vi "Actor Core.vi"(8 "error in":errorcluster, 11 "New Project Wizard in":refnum<class "Update Project Wizard.lvclass">) -> (0 "error out":errorcluster, 3 "Actor out":refnum<class "Actor.lvclass">)   [LabVIEW 2013, in "SET Project Editor.lvlib" / "Update Project Wizard.lvclass"]
doc: "(<B>Filename</B>: Actor Framework.lvlib:Actor.lvclass:Actor Core.vi)\n\nReceives messages to the actor, reacts to them, and initiates any error handling that may shut the actor down.\n\nDescendant classes may override this VI to append parallel tasks for the actor to complete while it handles messages. Overrides use the Call Parent Method node."
uses:
  Update Project Wizard.lvclass
  <vilib>/ActorFramework/Actor/Actor.lvclass
  <vilib>/ActorFramework/Actor/Actor.lvclass/Actor.ctl
  <vilib>/ActorFramework/Message Enqueuer/Message Enqueuer.lvclass/Message Enqueuer.ctl
  Update Project Wizard.lvclass/Update Project Wizard.ctl
  lib/printf/messages/General/LV_Printf Msg.lvclass/LV_Printf Msg.ctl
  UI Wizard/UI Wizard.lvclass
  lib/printf/messages/General/Read Message.vi
  <vilib>/ActorFramework/Message Enqueuer/Init from Existing Queue.vi
  <vilib>/ActorFramework/Message Enqueuer/Enqueue.vi
  <vilib>/ActorFramework/Message Priority Queue/Priority Enqueue.vi
  <vilib>/ActorFramework/Message Enqueuer/Message Enqueuer.lvclass
  <vilib>/ActorFramework/Stop Msg/Stop Msg.lvclass
  UI Wizard Messages/Extract Project Strings Msg/Extract Project Strings Msg.lvclass
  UI Wizard Messages/Apply Changes Msg/Apply Changes Msg.lvclass
  lib/printf/Core/LV_Printf Core.lvclass
  lib/printf/messages/General/LV_Printf Msg.lvclass
panel:
  in  "Tab Control":enum32{"Page 1", "Page 2"}(tab)
  in  "Next1":bool
  out "ProjectName":string
  in  "Cancel1":bool
  in  "VI Selector":i32(listbox)
  in  "RTM Selector":i32(listbox)
  out "Status":string
  in  "Prev2":bool
  in  "Finish":bool
  # "Update Project Wizard"
  # "Select VIs"
  # "Select Run-Time Menus"
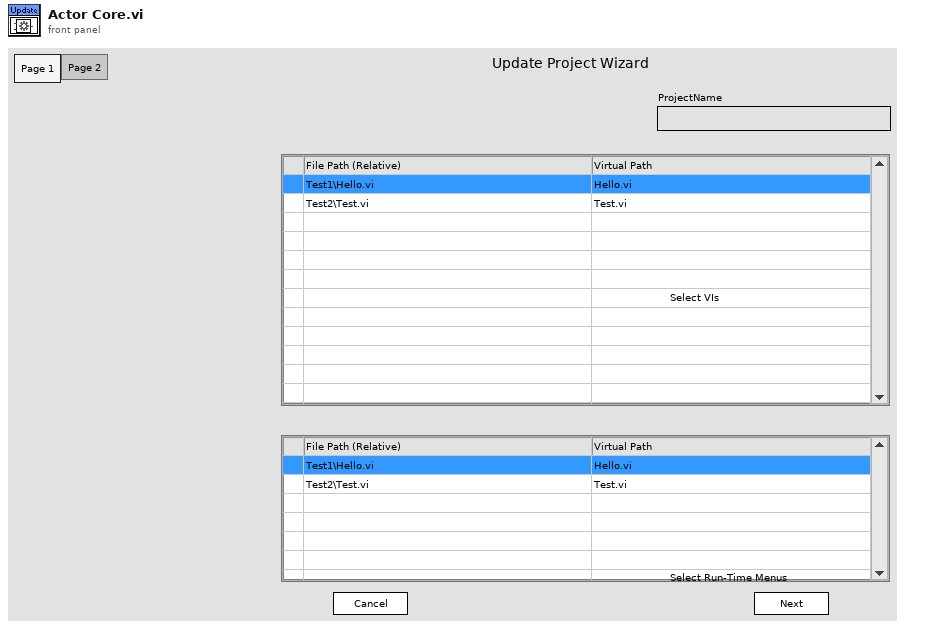
[diagram p1: front panel]
types:
  T1 = typedef "LVPoint32TypeDef.ctl" = cluster{"Horizontal":i32, "Vertical":i32}
  T2 = typedef "LVRowAndColumnTypeDef.ctl" = cluster{"Row":i32, "Column":i32}
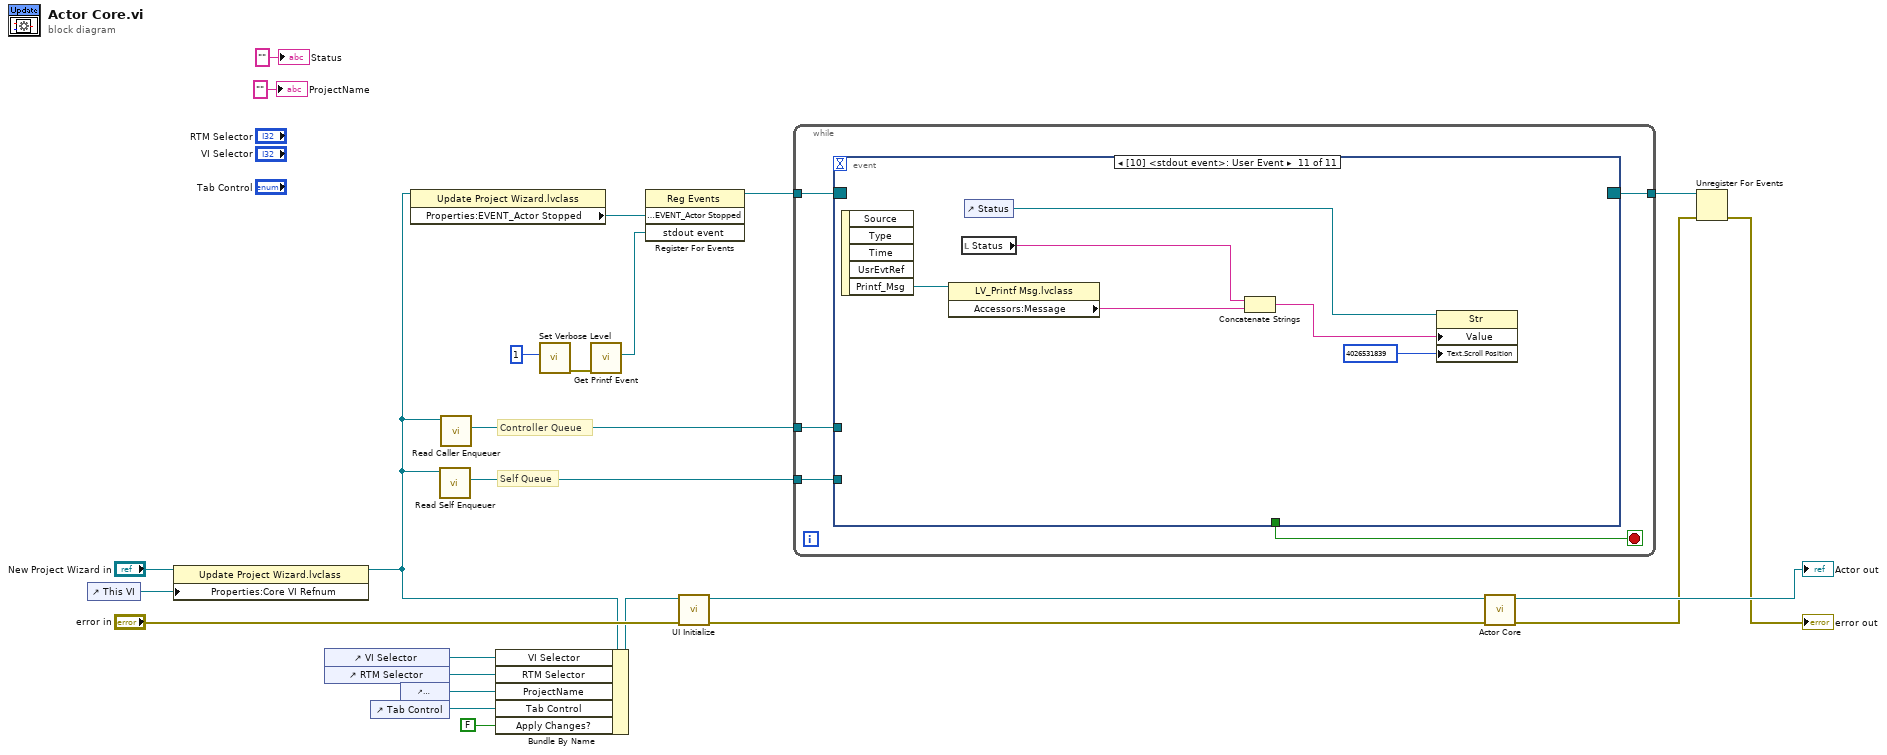
[diagram p0: block diagram]
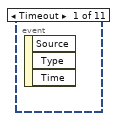
[diagram p2: hidden frame]
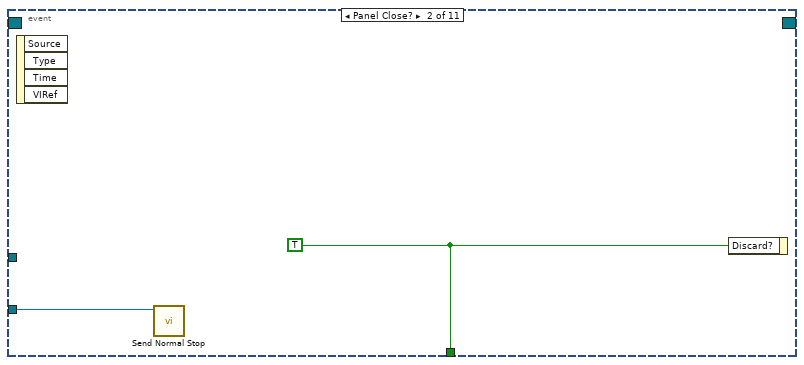
[diagram p3: hidden frame]
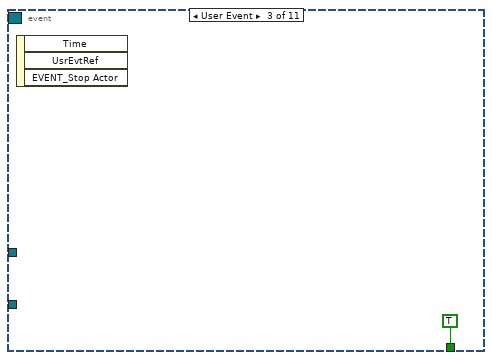
[diagram p4: hidden frame]
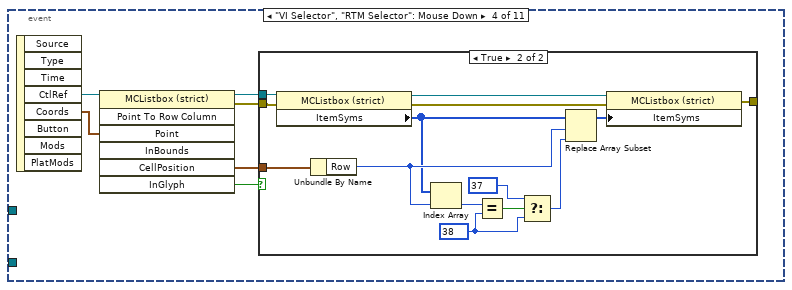
[diagram p5: hidden frame]
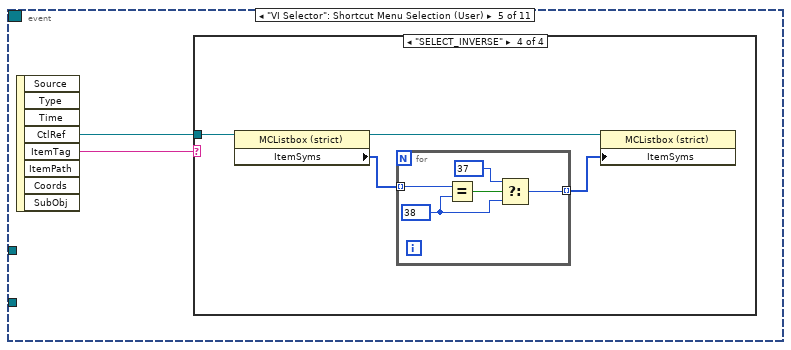
[diagram p7: hidden frame]
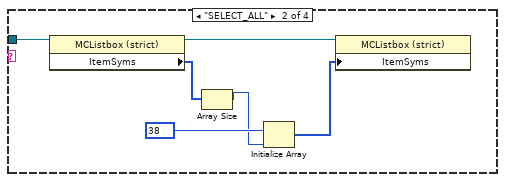
[diagram p9: hidden frame]
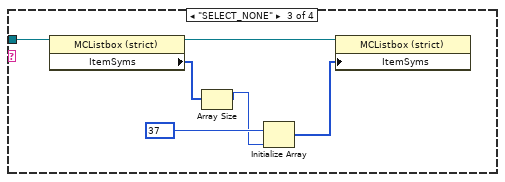
[diagram p10: hidden frame]
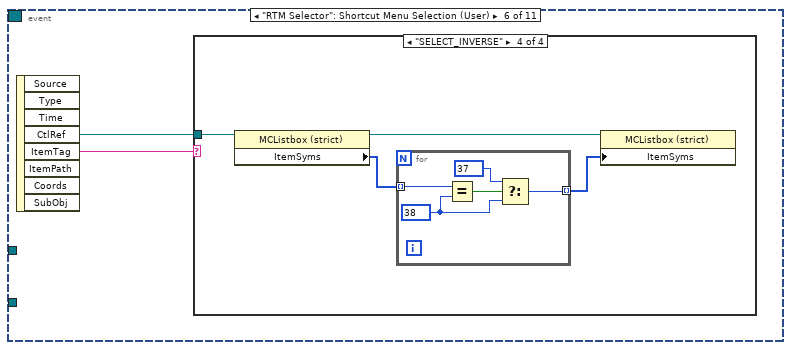
[diagram p11: hidden frame]
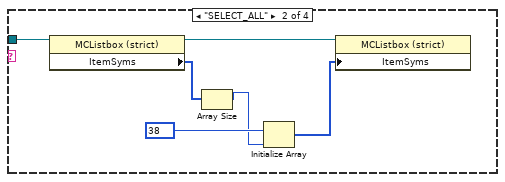
[diagram p13: hidden frame]
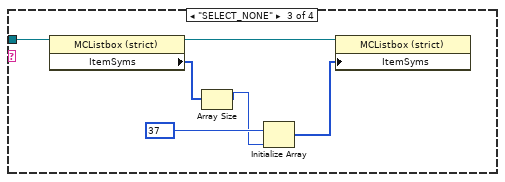
[diagram p14: hidden frame]
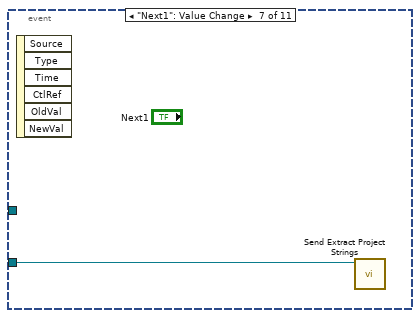
[diagram p15: hidden frame]
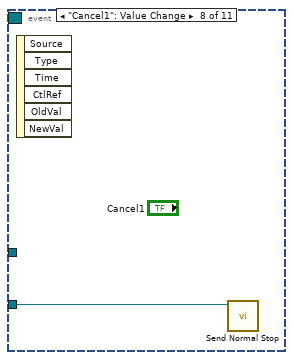
[diagram p16: hidden frame]
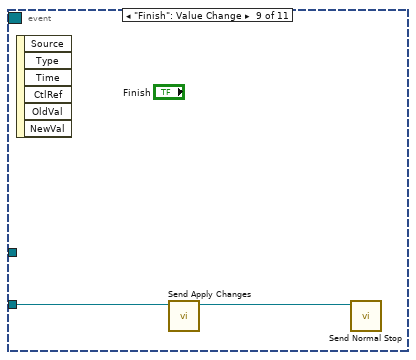
[diagram p17: hidden frame]
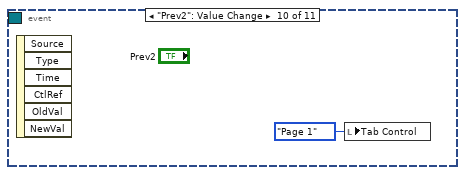
[diagram p18: hidden frame]
diagram:
  # "Controller Queue"
  # "Self Queue"
  n1 = control-ref of="This VI"() -> (w17:refnum<vi>)
  n2 = property class="Update Project Wizard.lvclass"(reference="New Project Wizard in", "Properties:Core VI Refnum"=w17) -> (reference out=w9:refnum<class "Update Project Wizard.lvclass">)  [unwired: 1 in, 1 out]
  n3 = control-ref of="VI Selector"() -> (w7:refnum<vi>)
  n4 = control-ref of="RTM Selector"() -> (w6:refnum<vi>)
  n5 = control-ref of="Tab Control"() -> (w4:refnum<vi>)
  n6 = control-ref of="ProjectName"() -> (w5:refnum<vi>)
  n7 = property class="Update Project Wizard.lvclass"(reference=w9) -> ("Properties:EVENT_Actor Stopped"=w24:refnum<user-event>)  [unwired: 1 in, 2 out]
  n8 = call <vilib>:"Read Self Enqueuer.vi"("Actor"=w9) -> ("Self Enqueuer"=w22:refnum<class "Message Enqueuer.lvclass">)  [unwired: 10 in]
  n9 = call <vilib>:"Read Caller Enqueuer.vi"("Actor"=w9) -> ("Caller Enqueuer"=w23:refnum<class "Message Enqueuer.lvclass">)  [unwired: 10 in]
  n10 = Bundle By Name(cluster=w9, "VI Selector"=w7, "RTM Selector"=w6, "ProjectName"=w5, "Tab Control"=w4, "Apply Changes?"=FALSE) -> (w8:refnum<class "Update Project Wizard.lvclass">)
  n11 = call "Set Verbose Level.vi"("Verbose Level"=1) -> ("error out"=w11:errorcluster)  [unwired: 10 in]
  n12 = call "Get Printf Event.vi"("error in (no error)"=w11) -> ("stdout event"=w10:refnum<user-event>)  [unwired: 8 in, 2 out]
  n13 = register-events(w24, w10) -> (reference out=w12:refnum<event-registration>)  [unwired: 2 in, 1 out]
  n14 = call-dynamic "UI Initialize.vi"("error in (no error)"="error in", "New Project Wizard in"=w8) -> ("error out"=w15:errorcluster, "New Project Wizard out"=w16:refnum<class "Update Project Wizard.lvclass">)  [unwired: 8 in]
  n15 = while {
    tunnel: w12 -> [w29]
    tunnel: [w28] -> w21
    tunnel: w22 -> [w27]
    tunnel: w23 -> [w26]
    stop <- w30 stop-if-true
    n16 = event shown="[10] <stdout event>: User Event" {
      selector: w29 -> [_ _ _ _ _ _ _ _ _ _ _]
      dyn-events: [_ _ _ _ _ _ _ _ _ _ _] -> w28
      timeout: _ -> [_ _ _ _ _ _ _ _ _ _ _]
      tunnel: [_ w32 TRUE ("Discard?") _ _ _ _ _ _ _ _] -> w30
      tunnel: w27 -> [_ w31 _ _ _ _ w101 w102 w104 _ _]
      tunnel: w26 -> [_ _ _ _ _ _ _ _ _ _ _]
      event Timeout {
        n17 = event-data() -> ()  [unwired: 1 in, 3 out]
      }
      event Panel Close? {
        w32 = TRUE ("Discard?")
        n18 = event-data() -> ()  [unwired: 1 in, 4 out]
        n19 = call <vilib>:"Send Normal Stop.vi"("Message Enqueuer"=w31) -> ()  [unwired: 10 in, 1 out]
        n20 = event-data("Discard?"=w32) -> ()  [unwired: 1 in, 1 out]
      }
      event User Event {
        n21 = event-data() -> ()  [unwired: 1 in, 3 out]
      }
      event "VI Selector", "RTM Selector": Mouse Down {
        n22 = event-data() -> ("CtlRef"=w35:refnum<vi>, "Coords"=w34:T1)  [unwired: 1 in, 6 out]
        n23 = invoke class="MCListbox (strict)" method="Point To Row Column"(reference=w35, "Point"=w34) -> (reference out=w37:refnum<vi>, error out=w38:errorcluster, "CellPosition"=w39:T2, "InGlyph"=w36:bool)  [unwired: 5 in, 3 out]
        n24 = case shown="True" w36 {
          tunnel: w39 -> [_ w54]
          tunnel: w38 -> [w40 w53]
          tunnel: [w40 w50] -> _
          tunnel: w37 -> [_ w49]
          frame False {
          }
          frame True {
            w45 = 38
            n25 = property on="Property Node" class="MCListbox (strict)"(reference=w49, error in=w53) -> (reference out=w48:refnum<vi>, error out=w52:errorcluster, "ItemSyms"=w42:i32[])
            n26 = Unbundle By Name(w54) -> ("Row"=w43:i32)
            n27 = Index Array(array=w42, index=w43) -> (element=w47:i32)
            n28 = Equal?(x=w47, y=w45) -> (x = y?=w46:bool)
            n29 = Select(t=37, s=w46, f=w45) -> (s? t:f=w44:i32)
            n30 = Replace Array Subset(array=w42, new element=w44, index=w43) -> (w51:i32[])
            n31 = property on="Property Node" class="MCListbox (strict)"(reference=w48, error in=w52, "ItemSyms"=w51) -> (error out=w50:errorcluster)  [unwired: 1 out]
          }
        }
      }
      event "VI Selector": Shortcut Menu Selection (User) {
        n32 = event-data() -> ("CtlRef"=w55:refnum<vi>, "ItemTag"=w56:string)  [unwired: 1 in, 6 out]
        n33 = case shown="\"SELECT_INVERSE\"" w56 {
          tunnel: w55 -> [_ w62 w68 w72]
          frame "False", Default {
          }
          frame "SELECT_ALL" {
            n34 = property class="MCListbox (strict)"(reference=w62) -> (reference out=w57:refnum<vi>, "ItemSyms"=w61:i32[])  [unwired: 1 in, 1 out]
            n35 = Array Size(array=w61) -> (size(s)=w59:i32)
            n36 = Initialize Array(38, w59) -> (w58:i32[])
            n37 = property class="MCListbox (strict)"(reference=w57, "ItemSyms"=w58) -> ()  [unwired: 1 in, 2 out]
          }
          frame "SELECT_NONE" {
            n38 = property class="MCListbox (strict)"(reference=w68) -> (reference out=w63:refnum<vi>, "ItemSyms"=w67:i32[])  [unwired: 1 in, 1 out]
            n39 = Array Size(array=w67) -> (size(s)=w65:i32)
            n40 = Initialize Array(37, w65) -> (w64:i32[])
            n41 = property class="MCListbox (strict)"(reference=w63, "ItemSyms"=w64) -> ()  [unwired: 1 in, 2 out]
          }
          frame "SELECT_INVERSE" {
            n42 = property class="MCListbox (strict)"(reference=w72) -> (reference out=w71:refnum<vi>, "ItemSyms"=w70:i32[])  [unwired: 1 in, 1 out]
            n43 = for {
              tunnel: w70 -> [w77] mode=indexing
              tunnel: [w73] -> w69 mode=indexing
              w74 = 38
              n44 = Equal?(x=w77, y=w74) -> (x = y?=w76:bool)
              n45 = Select(t=37, s=w76, f=w74) -> (s? t:f=w73:i32)
            }
            n46 = property class="MCListbox (strict)"(reference=w71, "ItemSyms"=w69) -> ()  [unwired: 1 in, 2 out]
          }
        }
      }
      event "RTM Selector": Shortcut Menu Selection (User) {
        n47 = event-data() -> ("CtlRef"=w78:refnum<vi>, "ItemTag"=w79:string)  [unwired: 1 in, 6 out]
        n48 = case shown="\"SELECT_INVERSE\"" w79 {
          tunnel: w78 -> [_ w85 w91 w95]
          frame "False", Default {
          }
          frame "SELECT_ALL" {
            n49 = property class="MCListbox (strict)"(reference=w85) -> (reference out=w80:refnum<vi>, "ItemSyms"=w84:i32[])  [unwired: 1 in, 1 out]
            n50 = Array Size(array=w84) -> (size(s)=w82:i32)
            n51 = Initialize Array(38, w82) -> (w81:i32[])
            n52 = property class="MCListbox (strict)"(reference=w80, "ItemSyms"=w81) -> ()  [unwired: 1 in, 2 out]
          }
          frame "SELECT_NONE" {
            n53 = property class="MCListbox (strict)"(reference=w91) -> (reference out=w86:refnum<vi>, "ItemSyms"=w90:i32[])  [unwired: 1 in, 1 out]
            n54 = Array Size(array=w90) -> (size(s)=w88:i32)
            n55 = Initialize Array(37, w88) -> (w87:i32[])
            n56 = property class="MCListbox (strict)"(reference=w86, "ItemSyms"=w87) -> ()  [unwired: 1 in, 2 out]
          }
          frame "SELECT_INVERSE" {
            n57 = property class="MCListbox (strict)"(reference=w95) -> (reference out=w94:refnum<vi>, "ItemSyms"=w93:i32[])  [unwired: 1 in, 1 out]
            n58 = for {
              tunnel: w93 -> [w100] mode=indexing
              tunnel: [w96] -> w92 mode=indexing
              w97 = 38
              n59 = Equal?(x=w100, y=w97) -> (x = y?=w99:bool)
              n60 = Select(t=37, s=w99, f=w97) -> (s? t:f=w96:i32)
            }
            n61 = property class="MCListbox (strict)"(reference=w94, "ItemSyms"=w92) -> ()  [unwired: 1 in, 2 out]
          }
        }
      }
      event "Next1": Value Change {
        n62 = event-data() -> ()  [unwired: 1 in, 6 out]
        n63 = call "Send Extract Project Strings.vi"("Message Enqueuer"=w101) -> ()  [unwired: 9 in, 2 out]
      }
      event "Cancel1": Value Change {
        n64 = event-data() -> ()  [unwired: 1 in, 6 out]
        n65 = call <vilib>:"Send Normal Stop.vi"("Message Enqueuer"=w102) -> ()  [unwired: 10 in, 1 out]
      }
      event "Finish": Value Change {
        n66 = event-data() -> ()  [unwired: 1 in, 6 out]
        n67 = call "Send Apply Changes.vi"("Message Enqueuer"=w104) -> ("Message Enqueuer out"=w103:refnum<class "Message Enqueuer.lvclass">)  [unwired: 9 in, 1 out]
        n68 = call <vilib>:"Send Normal Stop.vi"("Message Enqueuer"=w103) -> ()  [unwired: 10 in, 1 out]
      }
      event "Prev2": Value Change {
        n69 = event-data() -> ()  [unwired: 1 in, 6 out]
        n70 = local write "Tab Control"(enum32{"Page 1", "Page 2"}."Page 1" ("Tab Control")) -> ()
      }
      event User Event {
        n71 = event-data() -> ("Printf_Msg"=w109:refnum<class "LV_Printf Msg.lvclass">)  [unwired: 1 in, 4 out]
        n72 = property class="LV_Printf Msg.lvclass"(reference=w109) -> ("Accessors:Message"=w107:string)  [unwired: 1 in, 2 out]
        n73 = local read "Status"() -> (w108:string)
        n74 = control-ref of="Status"() -> (w111:refnum<vi>)
        n75 = Concatenate Strings(w108, w107) -> (w106:string)
        n76 = property class="Str"(reference=w111, "Value"=w106, "Text.Scroll Position"=u32 4026531839) -> ()  [unwired: 1 in, 2 out]
      }
    }
  }
  n77 = call-parent "Actor Core.vi"("error in"=w15, "Actor in"=w16) -> ("error out"=w20:errorcluster, "Actor out"=→"Actor out":refnum<class "Actor.lvclass">)  [unwired: 8 in]
  n78 = Unregister For Events(event registration refnum=w21, error in=w20) -> (error out=→"error out":errorcluster)
  "ProjectName" <- "" ("ProjectName")
  "Status" <- "" ("Status")
